vi "dashWrite_ShootDualTalonSRX.vi"   [LabVIEW 2019, in "ShootDualTalonSRX_Motor_Pair.lvlib"]
doc: "This VI is called for each TeleOp packet received from the DS where the robot is not disabled. It is often used to read from the joysticks and update I/O or to update setpoints for timed control loops. It should complete and return within 20 milliseconds or it may miss DS packets."
uses:
  ShootDualTalonSRX_Motor_Pair.lvlib
  globals_ShootDualTalonSRX.vi
  <vilib>/Rock Robotics/Network Tables/NT Write Boolean.vi
  <vilib>/Rock Robotics/Network Tables/NT Write Number.vi
  <vilib>/Rock Robotics/Network Tables/NT Write Numeric Array.vi
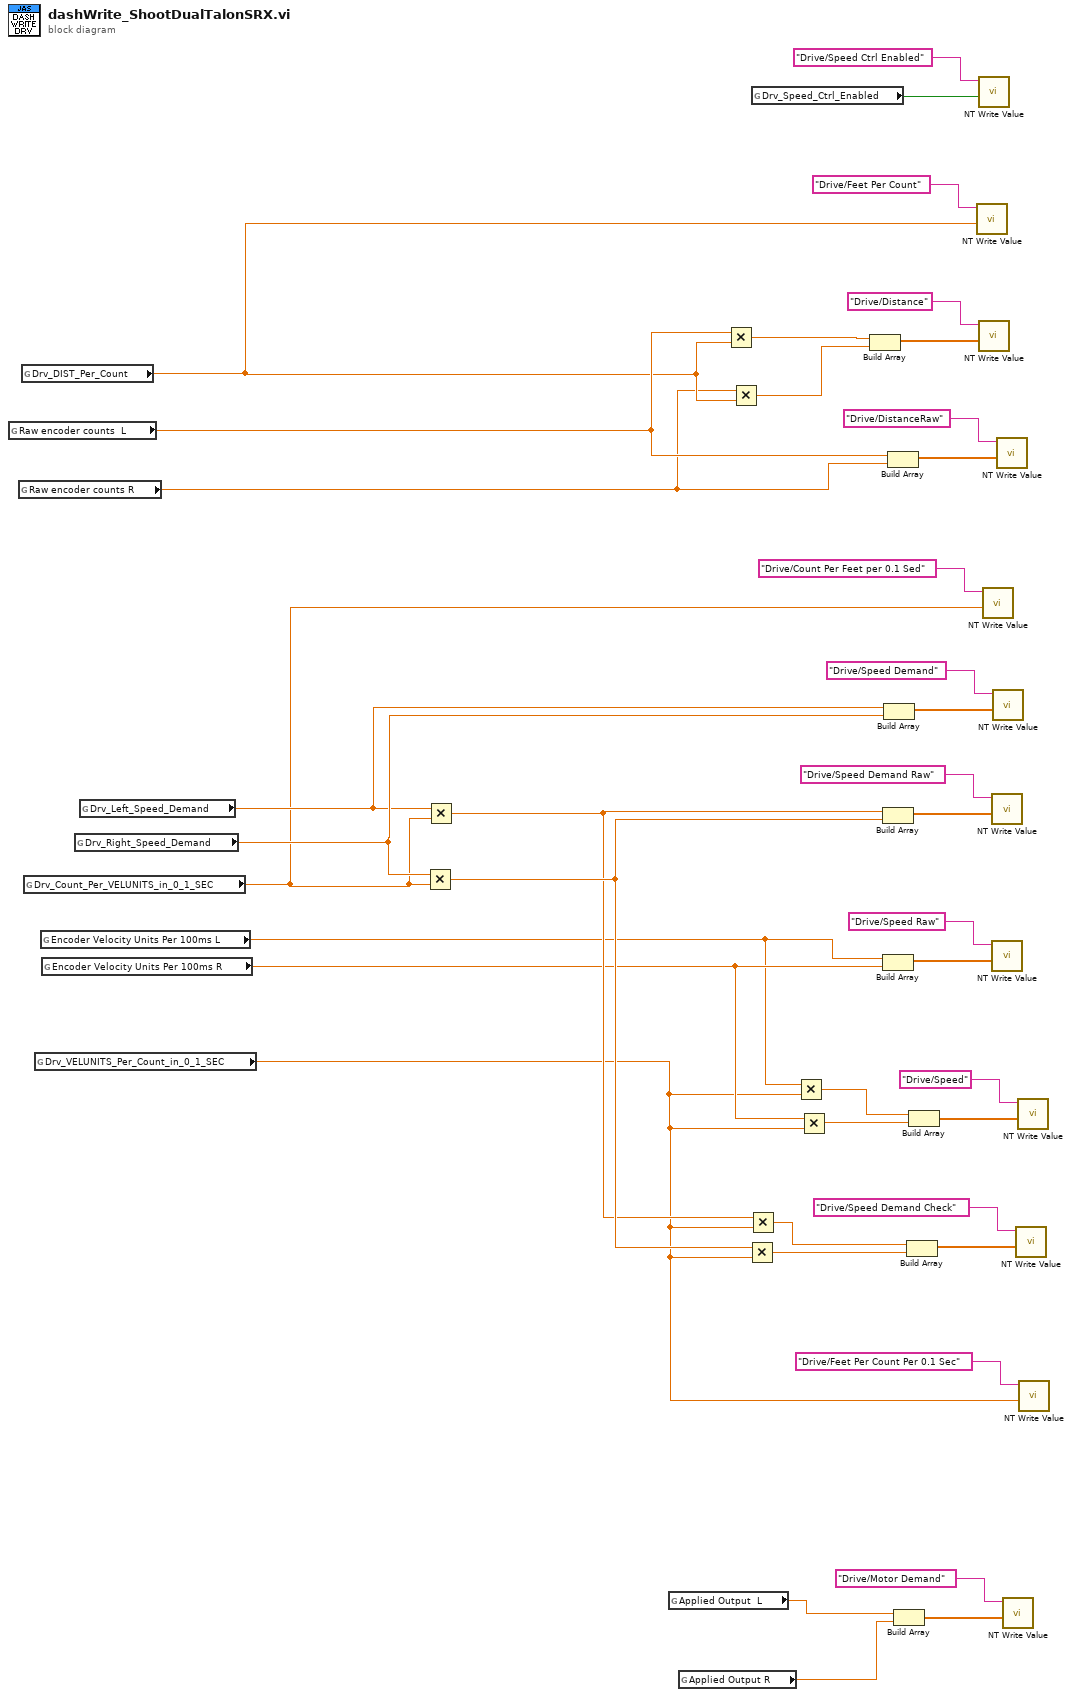
[diagram p0: block diagram]
diagram:
  n1 = global read "globals_ShootDualTalonSRX.vi" "Raw encoder counts  L"() -> (w6:dbl)
  n2 = global read "globals_ShootDualTalonSRX.vi" "Raw encoder counts R"() -> (w4:dbl)
  n3 = global read "globals_ShootDualTalonSRX.vi" "Drv_DIST_Per_Count"() -> (w5:dbl)
  n4 = global read "globals_ShootDualTalonSRX.vi" "Drv_Count_Per_VELUNITS_in_0_1_SEC"() -> (w10:dbl)
  n5 = global read "globals_ShootDualTalonSRX.vi" "Drv_VELUNITS_Per_Count_in_0_1_SEC"() -> (w1:dbl)
  n6 = global read "globals_ShootDualTalonSRX.vi" "Encoder Velocity Units Per 100ms L"() -> (w2:dbl)
  n7 = global read "globals_ShootDualTalonSRX.vi" "Encoder Velocity Units Per 100ms R"() -> (w3:dbl)
  n8 = global read "globals_ShootDualTalonSRX.vi" "Drv_Right_Speed_Demand"() -> (w33:dbl)
  n9 = global read "globals_ShootDualTalonSRX.vi" "Drv_Left_Speed_Demand"() -> (w32:dbl)
  n10 = Multiply(x=w33, y=w10) -> (x*y=w29:dbl)
  n11 = Multiply(x=w32, y=w10) -> (x*y=w28:dbl)
  n12 = global read "globals_ShootDualTalonSRX.vi" "Applied Output  L"() -> (w18:dbl)
  n13 = global read "globals_ShootDualTalonSRX.vi" "Applied Output R"() -> (w19:dbl)
  n14 = Multiply(x=w6, y=w5) -> (x*y=w7:dbl)
  n15 = Multiply(x=w4, y=w5) -> (x*y=w38:dbl)
  n16 = Multiply(x=w29, y=w1) -> (x*y=w15:dbl)
  n17 = Multiply(x=w28, y=w1) -> (x*y=w14:dbl)
  n18 = global read "globals_ShootDualTalonSRX.vi" "Drv_Speed_Ctrl_Enabled"() -> (w8:bool)
  n19 = Multiply(x=w2, y=w1) -> (x*y=w22:dbl)
  n20 = Multiply(x=w3, y=w1) -> (x*y=w23:dbl)
  n21 = Build Array(w7, w38) -> (w39:dbl[])
  n22 = Build Array(w28, w29) -> (w30:dbl[])
  n23 = Build Array(w2, w3) -> (w26:dbl[])
  n24 = Build Array(w32, w33) -> (w34:dbl[])
  n25 = Build Array(w6, w4) -> (w36:dbl[])
  n26 = Build Array(w18, w19) -> (w20:dbl[])
  n27 = Build Array(w14, w15) -> (w16:dbl[])
  n28 = Build Array(w22, w23) -> (w24:dbl[])
  n29 = call-poly <vilib>:"NT Write Value.vi"("Numeric"=w5, "Name"="Drive/Feet Per Count") -> ()  [unwired: 9 in, 1 out]
  n30 = call-poly <vilib>:"NT Write Value.vi"("Boolean"=w8, "Name"="Drive/Speed Ctrl Enabled") -> ()  [unwired: 9 in, 1 out]
  n31 = call-poly <vilib>:"NT Write Value.vi"("Numeric Array"=w39, "Name"="Drive/Distance") -> ()  [unwired: 9 in, 1 out]
  n32 = call-poly <vilib>:"NT Write Value.vi"("Numeric"=w10, "Name"="Drive/Count Per Feet per 0.1 Sed") -> ()  [unwired: 9 in, 1 out]
  n33 = call-poly <vilib>:"NT Write Value.vi"("Numeric Array"=w30, "Name"="Drive/Speed Demand Raw") -> ()  [unwired: 9 in, 1 out]
  n34 = call-poly <vilib>:"NT Write Value.vi"("Numeric Array"=w26, "Name"="Drive/Speed Raw") -> ()  [unwired: 9 in, 1 out]
  n35 = call-poly <vilib>:"NT Write Value.vi"("Numeric Array"=w34, "Name"="Drive/Speed Demand") -> ()  [unwired: 9 in, 1 out]
  n36 = call-poly <vilib>:"NT Write Value.vi"("Numeric Array"=w36, "Name"="Drive/DistanceRaw") -> ()  [unwired: 9 in, 1 out]
  n37 = call-poly <vilib>:"NT Write Value.vi"("Numeric Array"=w20, "Name"="Drive/Motor Demand") -> ()  [unwired: 9 in, 1 out]
  n38 = call-poly <vilib>:"NT Write Value.vi"("Numeric Array"=w16, "Name"="Drive/Speed Demand Check") -> ()  [unwired: 9 in, 1 out]
  n39 = call-poly <vilib>:"NT Write Value.vi"("Numeric Array"=w24, "Name"="Drive/Speed") -> ()  [unwired: 9 in, 1 out]
  n40 = call-poly <vilib>:"NT Write Value.vi"("Numeric"=w1, "Name"="Drive/Feet Per Count Per 0.1 Sec") -> ()  [unwired: 9 in, 1 out]
